vi "Loop_ACT.vi"() -> ()   [LabVIEW 2017, in "Claw_Rotation.lvlib"]
uses:
  Claw_Rotation.lvlib
  _SHARE ALL/TypeDef Share All/CLUSTER_TalonInput.ctl
  System Drivers/Phoenix-LabVIEW/Motor Controller/Controls/CTRE_Phoenix_MotorControl_ControlMode.ctl
  TypeDef/CLUSTER_PID.ctl
  _SHARE ALL/TypeDef Share All/CONTROL_PositonGraph.ctl
  CLUSTER_ACT_Lift Output.ctl
  _SHARE ALL/RoboRio Share All/SRX Share All/TypeDefs SRX/Cluster_SRX_Common Runtime Data.ctl
  _SHARE ALL/RoboRio Share All/SRX Share All/TypeDefs SRX/Cluster_SRX_Error Calculations.ctl
  _SHARE ALL/RoboRio Share All/SRX Share All/TypeDefs SRX/Cluster_SRX_Voltage Out Data.ctl
  _SHARE ALL/RoboRio Share All/SRX Share All/TypeDefs SRX/Cluster_SRX_Sensor Out Data.ctl
  _SHARE ALL/RoboRio Share All/SRX Share All/TypeDefs SRX/Cluster_SRX_F and R Limit Indicators.ctl
  Globals/Global_Device_IDs.vi
  _SHARE ALL/Global Share All/Global_STOP.vi
  Global_SM Write_Data Out.vi
  Global_ACT Write_Data Out.vi
panel:
  out "Rotation Output":T1 {"Common Runtime Data"."Temp" format="%.1f"; "Common Runtime Data"."Voltage"."Bus" format="%.3f"; "Common Runtime Data"."Voltage"."Output" format="%.3f"; "Common Runtime Data"."Voltage"."Percent" format="%.3f"; "Common Runtime Data"."Current" format="%.2f"}
  in  "Display Graph":bool
  out "Position Closed Loop Plots":T7
  out "Rotation Input":T8 {"Talon Mode" items=["PercentOutput"=0, "Position"=1, "Velocity"=2, "Current"=3, "Follower"=5, "MotionProfile"=6, "MotionMagic"=7, "MotionMagicArc"=8, "MotionProfileArc"=10, "Disabled"=15]}
  out "Cycle Time (S)":dbl format="%.3g"
  in  "Target Time(ms)":u32=50
  # "C"
  # "Units"
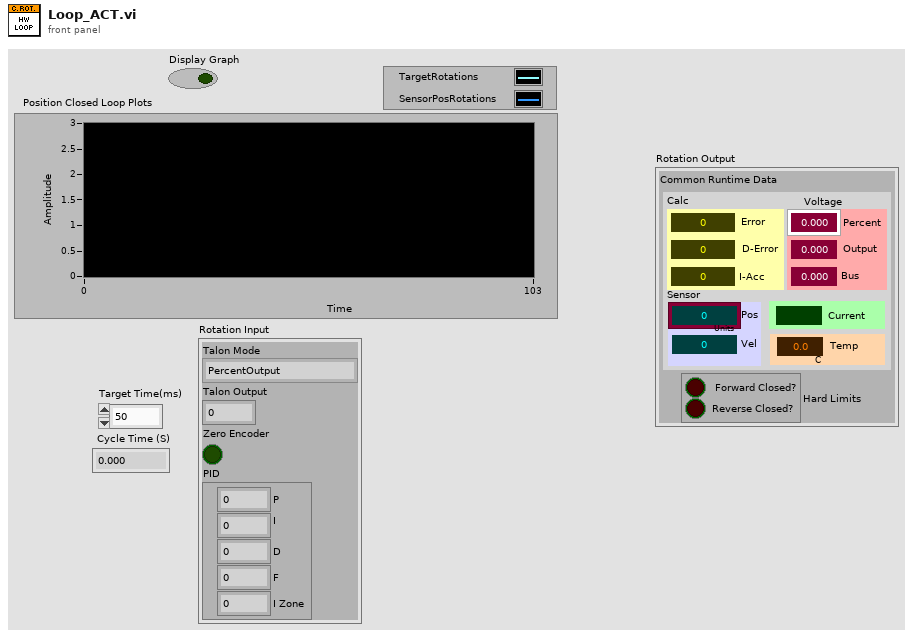
[diagram p1: front panel]
types:
  T1 = typedef "Claw_Rotation.lvlib/CLUSTER_ACT_Lift Output.ctl" = cluster{"Common Runtime Data":T2, "Hard Limits":T6}
  T2 = typedef "Cluster_SRX_Common Runtime Data.ctl" = cluster{"Calc":T3, "Voltage ":T4, "Sensor":T5, "Current":dbl, "Temp":dbl}
  T3 = typedef "Cluster_SRX_Error Calculations.ctl" = cluster{"Error":i32, "D-Error":dbl, "I-Acc":dbl}
  T4 = typedef "Cluster_SRX_Voltage Out Data.ctl" = cluster{"Percent":dbl, "Output":dbl, "Bus":dbl}
  T5 = typedef "Cluster_SRX_Sensor Out Data.ctl" = cluster{"Pos":i32, "Vel":i32}
  T6 = typedef "Cluster_SRX_F and R Limit Indicators.ctl" = cluster{"Forward Closed?":bool, "Reverse Closed?":bool}
  T7 = typedef "CONTROL_PositonGraph.ctl" = cluster{dbl, "Position (Raw Sensor Units)":i32}
  T8 = typedef "CLUSTER_TalonInput.ctl" = cluster{"Talon Mode":T9, "Talon Output":dbl, "Zero Encoder":bool, "PID":T10}
  T9 = typedef "CTRE_Phoenix_MotorControl_ControlMode.ctl" = u16
  T10 = typedef "CLUSTER_PID.ctl" = cluster{"P":dbl, "I":dbl, "D":dbl, "F":dbl, "I Zone":dbl}
  T11 = typedef "CLUSTER_Talon_Setup.ctl" = cluster{"Open Data":T12, "Current Config Data":T13, "Sensor Config":T14, "Hard Limits":T16, "Motion Magic Config Data":T18, "PIDF":T19, "Maximum Integral Accumulator Value":dbl, "AllowableClosedLoop":i32, "Limits":T20, "Output Config":T21}
  T12 = typedef "Cluster_SRX_OPEN Data.ctl" = cluster{"SRX ID":u8, "Invert Output":bool}
  T13 = typedef "Cluster_SRX_Current Config.ctl" = cluster{"Enable Current Limit?":bool, "Peak Current (Amps)":i32, "Peak Current Maximum Duration (ms)":i32, "Continuous Current Limit (Amps)":i32}
  T14 = typedef "Cluster_SRX_Sensor Config.ctl" = cluster{"Feedback Device":T15, "PhaseSensor":bool}
  T15 = typedef "CTRE_Phoenix_MotorControl_FeedbackDevice.ctl" = i8
  T16 = typedef "Cluster_SRX_Config Hard Limits.ctl" = cluster{"Fwd Enable":bool, "Rev Enable":bool, "Fwd NO-NC":T17, "Rev NO-NC":T17}
  T17 = typedef "CTRE_Phoenix_MotorControl_LimitSwitchNormal.ctl" = enum16{"Normally Open", "Normally Closed", "Disabled"}
  T18 = typedef "Cluster_SRX_Motion Magic Config Data.ctl" = cluster{"Cruise Velocity":i32, "Acceleration":i32}
  T19 = typedef "Cluster_SRX_PIDF.ctl" = cluster{"P":dbl, "I":dbl, "D":dbl, "F":dbl, "I Zone":dbl}
  T20 = typedef "Cluster_SRX_Config Soft Limits.ctl" = cluster{"Max":i32, "Min":i32, "Max Enable":bool, "Min Enable":bool}
  T21 = typedef "Cluster_SRX_Config Voltage Output.ctl" = cluster{"Invert?":bool, "Neutral Mode":T22, "Deadband (-1to1)":dbl, "Ramp Time Off to Full (S)":dbl, "Peak  (-1to1)":T23, "Nominal  (-1to1)":T23}
  T22 = typedef "CTRE_Phoenix_MotorControl_NeutralMode.ctl" = enum8{"EEPROMSetting", "Override to Coast", "Override to Brake"}
  T23 = typedef "Cluster_SRX_Forward and Reverse.ctl" = cluster{"Forward":dbl, "Reverse":dbl}
  T24 = typedef "WPI_MotorControlDeviceRef.ctl" = cluster{"DeviceStatus":errorcluster, "Type":T25, "PWM":cluster{"PWM Channel":T26, "DeadBand":T27}, "CAN":cluster{"Device Number":u8, "SetOutput VI Ref":variant, "GetOutput VI Ref":variant, "Enable VI Ref":variant, "Disable VI Ref":variant, "Data":variant}, "Invert":bool, "DIO PWM":cluster{"PWM \"Enable\" Channel":T26, "DIOChannel":T28, "PWM Rate":dbl}}
  T25 = typedef "WPI_MotorControlType.ctl" = enum16{"PWM", "CAN", "DIO PWM"}
  T26 = typedef "FPGA_DIOPWMChannel.ctl" = enum8{"PWM 0", "PWM 1", "PWM 2", "PWM 3", "PWM 4", "PWM 5", "PWM 6", "PWM 7", "PWM 8", "PWM 9", "PWM MXP 0", "PWM MXP 1", "PWM MXP 2", "PWM MXP 3", "PWM MXP 4", "PWM MXP 5", "PWM MXP 6", "PWM MXP 7", "PWM MXP 8", "PWM MXP 9", "Invalid"}
  T27 = typedef "WPI_PWMDeadband.ctl" = cluster{"Name":string, "maxPositivePwm":i32, "minPositivePwm":i32, "centerPwm":i32, "maxNegativePwm":i32, "minNegativePwm":i32, "angularRange":u16}
  T28 = typedef "FPGA_DIOChannel.ctl" = enum8{"DIO 0", "DIO 1", "DIO 2", "DIO 3", "DIO 4", "DIO 5", "DIO 6", "DIO 7", "DIO 8", "DIO 9", "DIO MXP 0", "DIO MXP 1", "DIO MXP 2", "DIO MXP 3", "DIO MXP 4", "DIO MXP 5", "DIO MXP 6", "DIO MXP 7", "DIO MXP 8", "DIO MXP 9", "DIO MXP 10", "DIO MXP 11", "DIO MXP 12", "DIO MXP 13", "DIO MXP 14", "DIO MXP 15", "SPI Port CS1", "SPI Port CS2", "SPI Port CS3", "SPI Port MISO", "SPI Port MOSI", "Invalid"}
  T29 = cluster{"PhoenixMotorControlDevRef":T24, "Claw Rotation Output":T1, "Claw Rotation Input":T8, "Target Time(ms)":u32, "Current Time":timestamp, "Previous Time":timestamp, "Cycle Time (S)":dbl, "Last PID":T10}
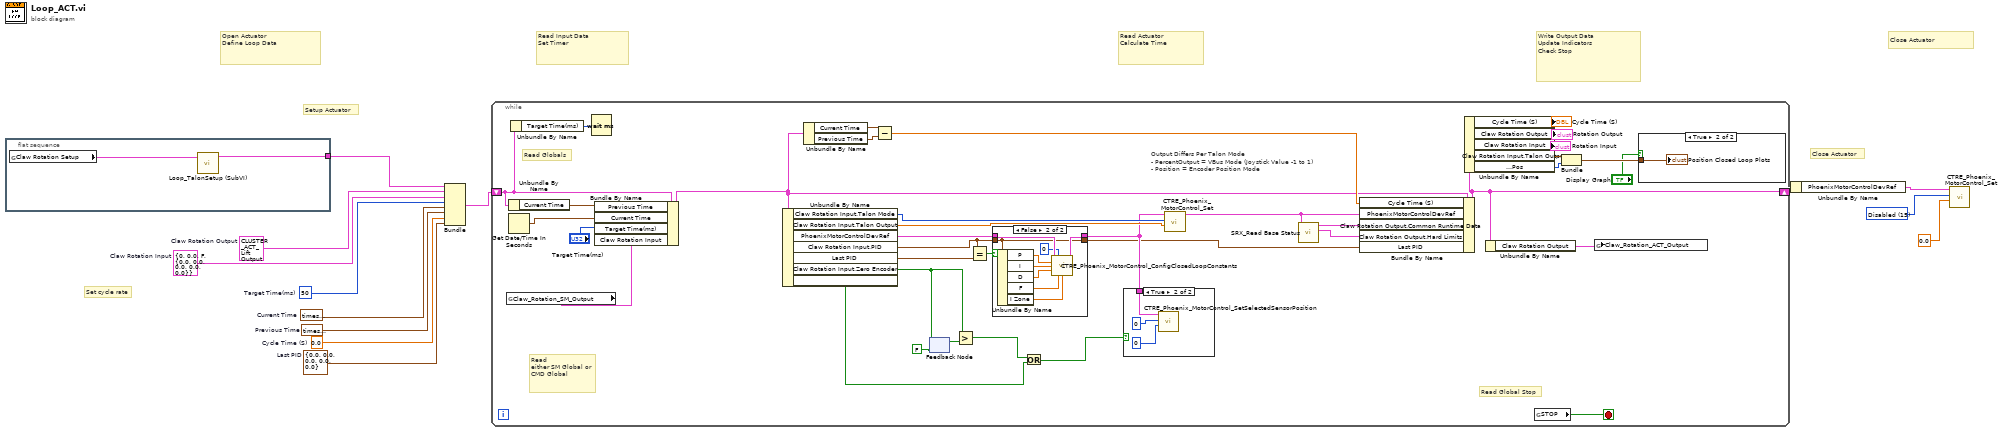
[diagram p0: block diagram]
diagram:
  w1 = T1 {"Common Runtime Data"={"Calc"={"Error"=0, "D-Error"=0.0, "I-Acc"=0.0}, "Voltage "={"Percent"=0.0, "Output"=0.0, "Bus"=0.0}, "Sensor"={"Pos"=0, "Vel"=0}, "Current"=0.0, "Temp"=0.0}, "Hard Limits"={"Forward Closed?"=FALSE, "Reverse Closed?"=FALSE}}  # Claw Rotation Output
  w3 = T10 {"P"=0.0, "I"=0.0, "D"=0.0, "F"=0.0, "I Zone"=0.0}  # Last PID
  w5 = T9 15 items=["PercentOutput"=0, "Position"=1, "Velocity"=2, "Current"=3, "Follower"=5, "MotionProfile"=6, "MotionMagic"=7, "MotionMagicArc"=8, "MotionProfileArc"=10, "Disabled"=15] ("Control Mode")
  w7 = T8 {"Talon Mode"=0, "Talon Output"=0.0, "Zero Encoder"=FALSE, "PID"={"P"=0.0, "I"=0.0, "D"=0.0, "F"=0.0, "I Zone"=0.0}}  # Claw Rotation Input
  w8 = 0.0  # Cycle Time (S)
  w13 = timestamp(0 s since 1904-01-01)  # Previous Time
  w12 = timestamp(0 s since 1904-01-01)  # Current Time
  w11 = u32 50  # Target Time(ms)
  # "Close Actuator"
  # "Write Output Data\nUpdate Indicators\nCheck Stop"
  # "Read Actuator\nCalculate Time"
  # "Read Input Data\nSet Timer"
  # "Open Actuator\nDefine Loop Data"
  # "Set cycle rate"
  # "Close Actuator"
  # "Setup Actuator"
  n1 = flat-sequence {
    tunnel: [w15] -> w2
    frame #0 {
      n2 = global read "Global_Device_IDs.vi" "Claw Rotation Setup"() -> (w14:T11)
      n3 = call "Loop_TalonSetup (SubVI).vi"("Talon Setup"=w14) -> ("PhoenixMotorControlDevRef"=w15:T24)  [unwired: 10 in]
    }
  }
  n4 = Bundle("PhoenixMotorControlDevRef"=w2, "Claw Rotation Output"=w1, "Claw Rotation Input"=w7, "Target Time(ms)"=w11, "Current Time"=w12, "Previous Time"=w13, "Cycle Time (S)"=w8, "Last PID"=w3) -> (w10:T29)  [unwired: 1 in]
  n5 = while {
    shift-right: [w44] -> w9
    shift-left: w10 -> [w46]
    stop <- w52 stop-if-true
    # "Output Differs Per Talon Mode\n- PercentOutput = VBus Mode (Joystick Value -1 to 1)\n- Position = Encoder Position Mode"
    # "Read\neither SM Global or CMD Global"
    # "Read Globals"
    # "Read Global Stop"
    n6 = global read "Global_SM Write_Data Out.vi" "Claw_Rotation_SM_Output"() -> (w40:T8)
    n7 = Unbundle By Name(w46) -> ("Current Time"=w50:timestamp)
    n8 = Get Date/Time In Seconds() -> (seconds since 1Jan1904=w51:timestamp)
    n9 = Unbundle By Name(w46) -> ("Target Time(ms)"=w45:u32)
    n10 = Wait (ms)(milliseconds to wait=w45) -> ()  [unwired: 1 out]
    n11 = Bundle By Name(cluster=w46, "Previous Time"=w50, "Current Time"=w51, "Target Time(ms)"="Target Time(ms)", "Claw Rotation Input"=w40) -> (w33:T29)
    n12 = Unbundle By Name(w33) -> ("Claw Rotation Input.Talon Mode"=w39:T9, "Claw Rotation Input.Talon Output"=w38:dbl, "PhoenixMotorControlDevRef"=w32:T24, "Claw Rotation Input.PID"=w28:T10, "Last PID"=w29:T10, "Claw Rotation Input.Zero Encoder"=w24:bool, "Claw Rotation Output.Hard Limits.Forward Closed?"=w16:bool)
    n13 = Unbundle By Name(w33) -> ("Current Time"=w49:timestamp, "Previous Time"=w48:timestamp)
    n14 = Subtract(x=w49, y=w48) -> (x-y=w42:dbl)
    n15 = feedback #1(FALSE) -> (w25:bool)
    n16 = feedback-in #1(w24) -> ()
    n17 = Greater?(x=w24, y=w25) -> (0:w18:bool)
    n18 = Equal?(x=w28, y=w29) -> (x = y?=w27:bool)
    n19 = case shown="False" w27 {
      tunnel: w32 -> [w54 w63]
      tunnel: [w54 w62] -> w31
      tunnel: w28 -> [w53 w55]
      tunnel: [w53 w55] -> w20
      frame True {
      }
      frame False {
        n20 = Unbundle By Name(w55) -> ("P"=w60:dbl, "I"=w59:dbl, "D"=w58:dbl, "F"=w57:dbl, "I Zone"=w56:dbl)
        n21 = call "CTRE_Phoenix_MotorControl_ConfigClosedLoopConstants.vi"("PhoenixMotorControlDevRef"=w63, "slotIdx"=0, "P"=w60, "I"=w59, "D"=w58, "F"=w57, "I Zone"=w56) -> ("PhoenixMotorControlDevRef"=w62:T24)  [unwired: 7 in, 1 out]
      }
    }
    n22 = Or(x=w18, y=w16) -> (x .or. y?=w17:bool)
    n23 = case shown="True" w17 {
      tunnel: w31 -> [_ w67]
      frame False {
      }
      frame True {
        n24 = call "CTRE_Phoenix_MotorControl_SetSelectedSensorPosition.vi"("pidLoopIdx"=u32 0, "New Sensor Position"=0, "PhoenixMotorControlDevRef"=w67) -> ()  [unwired: 7 in, 2 out]
      }
    }
    n25 = call "CTRE_Phoenix_MotorControl_Set.vi"("Output"=w38, "Control Mode"=w39, "PhoenixMotorControlDevRef"=w31) -> ("PhoenixMotorControlDevRef"=w23:T24)  [unwired: 7 in, 1 out]
    n26 = call "SRX_Read Base Status.vi"("PhoenixMotorControlDevRef"=w23) -> ("Hard Limits Out"=w21:T6, "Common Runtime Data Out"=w22:T2)  [unwired: 8 in, 1 out]
    n27 = Bundle By Name(cluster=w33, "Cycle Time (S)"=w42, "PhoenixMotorControlDevRef"=w23, "Claw Rotation Output.Common Runtime Data"=w22, "Claw Rotation Output.Hard Limits"=w21, "Last PID"=w20) -> (w44:T29)
    n28 = Unbundle By Name(w44) -> ("Cycle Time (S)"=→"Cycle Time (S)":dbl, "Claw Rotation Output"=→"Rotation Output":T1, "Claw Rotation Input"=→"Rotation Input":T8, "Claw Rotation Input.Talon Output"=w36:dbl, "Claw Rotation Output.Common Runtime Data.Sensor.Pos"=w35:i32)
    n29 = Unbundle By Name(w44) -> ("Claw Rotation Output"=w41:T1)
    n30 = global read "Global_STOP.vi" "STOP"() -> (w52:bool)
    n31 = Bundle("Talon Output"=w36, "Pos"=w35) -> (w34:cluster{"Talon Output":dbl, "Pos":i32})  [unwired: 1 in]
    n32 = global write "Global_ACT Write_Data Out.vi" "Claw_Rotation_ACT_Output"(w41) -> ()
    n33 = case shown="True" "Display Graph" {
      tunnel: w34 -> [_ w64]
      frame False {
      }
      frame True {
        "Position Closed Loop Plots" <- w64
      }
    }
  }
  n34 = Unbundle By Name(w9) -> ("PhoenixMotorControlDevRef"=w6:T24)
  n35 = call "CTRE_Phoenix_MotorControl_Set.vi"("Output"=0.0, "Control Mode"=w5, "PhoenixMotorControlDevRef"=w6) -> ()  [unwired: 7 in, 2 out]
